vi "motors.vi"() -> (0 "Lift Motor 1":dbl, 1 "Front Right Motor":cluster{"Value":dbl, "Constant":dbl}, 2 "Front Left Motor":cluster{"Value":dbl, "Constant":dbl}, 3 "Back Left Motor":cluster{"Value":dbl, "Constant":dbl}, 4 "Lift Motor 2":dbl, 5 "Back Right Motor":cluster{"Value":dbl, "Constant":dbl}, 6 "Container Arm Motor":dbl, 7 "Center Motor":cluster{"Value":dbl, "Constant":dbl}, 8 "motor array":dbl[](array[numeric]))   [LabVIEW 2014]
uses:
  <vilib>/Rock Robotics/Network Tables/NT Read Numeric Array.vi
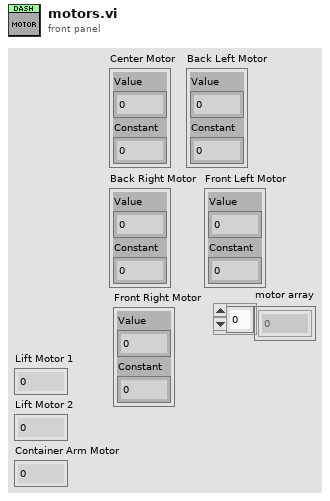
[diagram p1: front panel]
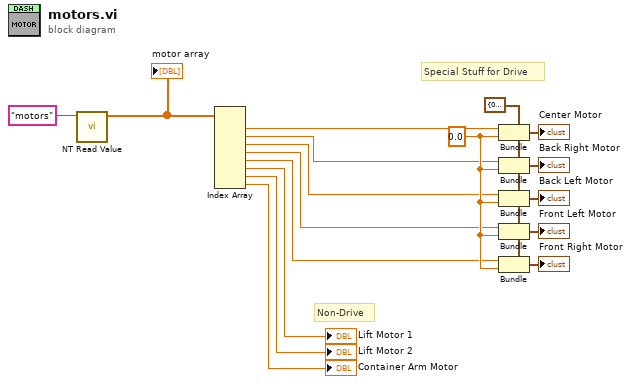
[diagram p0: block diagram]
diagram:
  w13 = 0.0
  w12 = cluster{"Value":dbl, "Constant":dbl} {"Value"=0.0, "Constant"=0.0} ("Center Wheel")
  # "Special Stuff for Drive"
  # "Non-Drive"
  n1 = call-poly <vilib>:"NT Read Value.vi"("Name"="motors") -> ("Numeric Array"=w1:dbl[])  [unwired: 9 in, 1 out]
  "motor array" <- w1
  n2 = Index Array(array=w1) -> (element #1=w2:dbl, element #2=w8:dbl, element #3=w11:dbl, element #4=w10:dbl, element #5=w9:dbl, element #6=→"Lift Motor 1":dbl, element #7=→"Lift Motor 2":dbl, element #8=→"Container Arm Motor":dbl)  [unwired: 8 in]
  n3 = Bundle(cluster=w12, "Value"=w2, "Constant"=w13) -> (→"Center Motor":cluster{"Value":dbl, "Constant":dbl})
  n4 = Bundle(cluster=w12, "Value"=w8, "Constant"=w13) -> (→"Back Right Motor":cluster{"Value":dbl, "Constant":dbl})
  n5 = Bundle(cluster=w12, "Value"=w11, "Constant"=w13) -> (→"Back Left Motor":cluster{"Value":dbl, "Constant":dbl})
  n6 = Bundle(cluster=w12, "Value"=w10, "Constant"=w13) -> (→"Front Left Motor":cluster{"Value":dbl, "Constant":dbl})
  n7 = Bundle(cluster=w12, "Value"=w9, "Constant"=w13) -> (→"Front Right Motor":cluster{"Value":dbl, "Constant":dbl})
